vi "AnalogInput.vi"(0 "Analog Input Channel":T1(ring), 3 "register values IN":u16[](array[numeric])) -> (7 "Analog Value":dbl, 10 "register values OUT":u16[](array[numeric]))   [LabVIEW 2025]
doc: "Returns floating point value of desired phys. \npanel analog input. Stackable, wire in series\nor parallel for multiple channel reading.\n\nINPUTS:\n 1. Analog input channel -- int 0-7 or auto\n configured enum AI-0 -> AI-7\n 2. Array of values read from MB server.\n int with dimension 8x1\n\nOUTPUTS:\n 1. Value from channel selected with input 1.\n floating point DBL\n 2. Array of values read from MB server.\n int with dimension 8x1. -- Direct passthrough\n of input 2"
panel:
  # "Read single analog input from array\n\nReturns floating point value of desired phys. \npanel analog input. Stackable, wire in series\nor parallel for multiple channel reading.\n\nINPUTS:\n  1. Analog input channel -- int 0-7 or auto\n      configured enum AI-0 -> AI-7\n   2. Array of values read from MB server.\n       int with dimension 8x1\n\nOUTPUTS:\n   1. Value from channel selected with input 1.\n       floating point DBL\n   2. Array of values read from MB server.\n       int with dimension 8x1. -- Direct passthrough\n       of input 2"
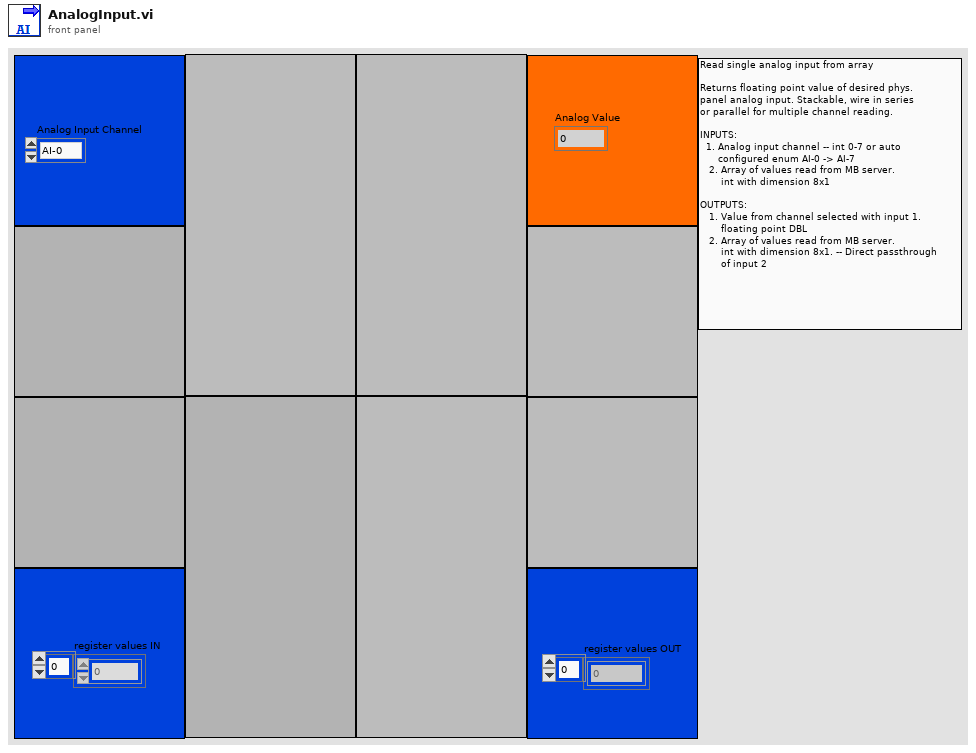
[diagram p1: front panel]
types:
  T1 = enum16{"AI-0", "AI-1", "AI-2", "AI-3", "AI-4", "AI-5", "AI-6", "AI-7"}
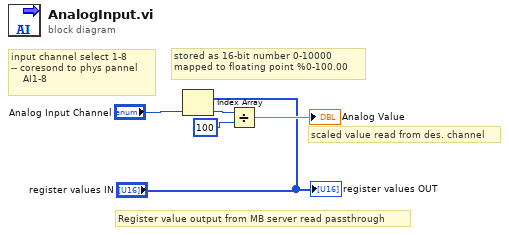
[diagram p0: block diagram]
diagram:
  # "scaled value read from des. channel"
  # "stored as 16-bit number 0-10000\nmapped to floating point %0-100.00"
  # "input channel select 1-8\n-- coresond to phys pannel\n    AI1-8"
  # "Register value output from MB server read passthrough"
  n1 = Index Array(array="register values IN", index="Analog Input Channel") -> (element=w3:u16)
  n2 = Divide(x=w3, y=u16 100) -> (x/y=→"Analog Value":dbl)
  "register values OUT" <- "register values IN"
